vi "create IFD.vi"(1 "Value/Offset":u32, 2 "Count":u32, 3 "TYPE":u16, 4 "TAG":u16) -> (0 "IFD entry":u16[](array[numeric]))   [LabVIEW 2012]
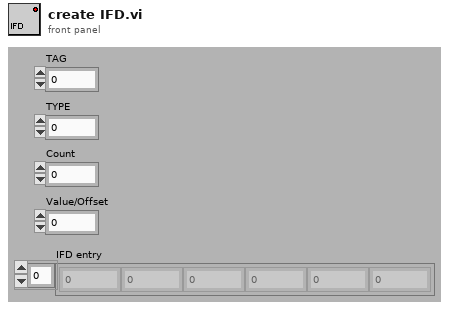
[diagram p1: front panel]
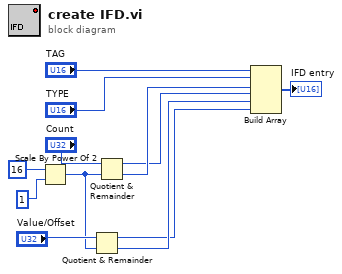
[diagram p0: block diagram]
diagram:
  n1 = Scale By Power Of 2(n=u32 16, x=u32 1) -> (x*2^n=w4:u32)
  n2 = Quotient & Remainder(x="Value/Offset", y=w4) -> (x-y*floor(x/y)=w2:u32, floor(x/y)=w3:u32)
  n3 = Quotient & Remainder(x="Count", y=w4) -> (x-y*floor(x/y)=w6:u32, floor(x/y)=w7:u32)
  n4 = Build Array("TAG", "TYPE", w7, w6, w3, w2) -> (→"IFD entry":u32[])
